vi "3458A Check Digitizing Process Status.vi"(5 "merge process exit error with main (True)":bool=TRUE, 7 "wait for exit (False)":bool, 8 "error in":errorcluster, 10 "channel id":i32, 11 "digitizer session in":T1 {"channels"."Range [Vpk]" min=0.0}) -> (0 "error out":errorcluster, 1 "proc error out":errorcluster, 2 "process exited?":bool, 3 "digitizer session out":T1 {"channels"."Range [Vpk]" min=0.0}, 4 "aux data out":T12, 6 "aux data valid?":bool)   [LabVIEW 2013, in "3458A Virtual Digitizer.lvlib"]
doc: "Checks execution status of digitizing process number 'channel id'. 'wait for exit' options specifies whether VI is just checking status or waits with timeout (3 seconds). If process exited and the 'wait for exit' is True the returned value from the process is returned in 'aux data out'. Exit status is returned in 'process exited' output. Once process exit value was returned, calling this VI will return error and invalid data!"
uses:
  3458A Virtual Digitizer.lvlib
  3458A Digitizer Session.ctl
  3458A Virtual Channel Config.ctl
  Counter/Counter Session.ctl
  Counter/Counter Type.ctl
  AWG/AWG Session.ctl
  AWG/AWG Type.ctl
  3458A Sync Mode.ctl
  3458A Idn Mode.ctl
  3458A Digitizing Low Levels/Configure/Sampling Mode.ctl
  3458A Digitizing Process Options.ctl
  3458A Data Packet.ctl
  3458A Aux Record Data.ctl
  3458A Digitizing Low Levels/Configure/Level Setup.ctl
  3458A Digitizing Low Levels/Configure/First Sample Trigger.ctl
  3458A Aperture Selection Mode.ctl
  Counter/Counter.lvlib
  AWG/AWG.lvlib
  3458A Digitizing Low Levels/3458A Digitizing Low Levels.lvlib
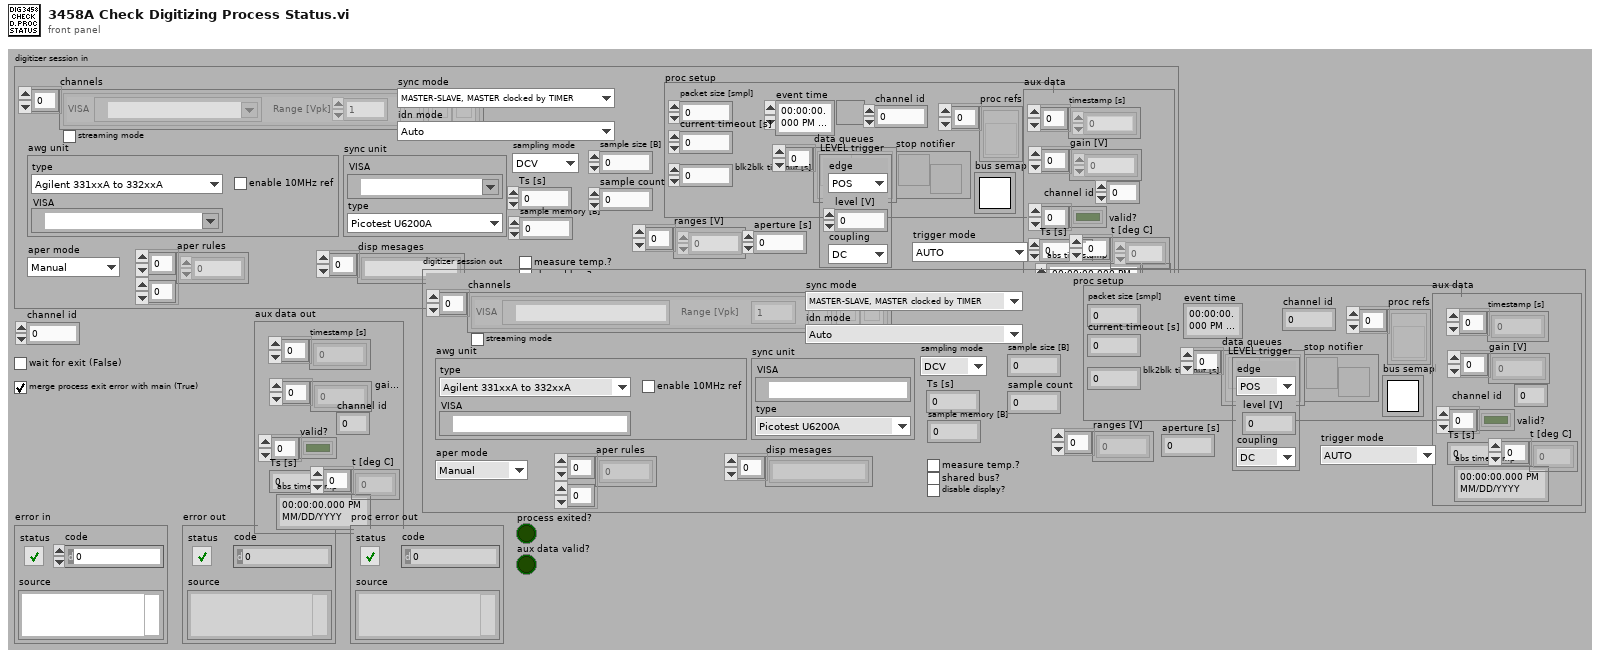
[diagram p1: front panel]
types:
  T1 = typedef "3458A Virtual Digitizer.lvlib/3458A Digitizer Session.ctl" = cluster{"channels":T2[], "sync unit":T3, "awg unit":T5, "sync mode":T7, "streaming mode":bool, "idn mode":T8, "sampling mode":T9, "Ts [s]":dbl, "sample memory [B]":i32, "proc setup":T10, "sample size [B]":i32, "sample count":i32, "aux data":T12, "ranges [V]":dbl[], "aperture [s]":dbl, "LEVEL trigger":T13, "trigger mode":T14, "measure temp.?":bool, "disp mesages":string[], "shared bus?":bool, "disable display?":bool, "aper mode":T15, "aper rules":dbl[][]}
  T2 = typedef "3458A Virtual Digitizer.lvlib/3458A Virtual Channel Config.ctl" = cluster{"VISA":refnum<visa-resource-name>, "Range [Vpk]":dbl, "btn clr":bool, "btn up":bool, "btn down":bool}
  T3 = typedef "Counter.lvlib/Counter Session.ctl" = cluster{"VISA":refnum<visa-resource-name>, "type":T4}
  T4 = typedef "Counter.lvlib/Counter Type.ctl" = enum16{"Picotest U6200A", "dummy"}
  T5 = typedef "AWG.lvlib/AWG Session.ctl" = cluster{"type":T6, "VISA":refnum<visa-resource-name>, "enable 10MHz ref":bool}
  T6 = typedef "AWG.lvlib/AWG Type.ctl" = enum16{"Agilent 331xxA to 332xxA", "Agilent 335xxA to 336xxA", "Tektronix AFG3101C", "dummy"}
  T7 = typedef "3458A Virtual Digitizer.lvlib/3458A Sync Mode.ctl" = enum16{"MASTER-SLAVE, MASTER clocked by TIMER", "MASTER-SLAVE, MASTER clocked by AWG", "ALL clocked by AWG", "MASTER-SLAVE, ALL clocked by TIMER", "ALL clocked by AWG with DFLL"}
  T8 = typedef "3458A Virtual Digitizer.lvlib/3458A Idn Mode.ctl" = enum16{"Auto", "Sequential (chn A, chn B, ...)", "From calibration string"}
  T9 = typedef "3458A Virtual Digitizer.lvlib/3458A Digitizing Low Levels.lvlib/Sampling Mode.ctl" = enum16{"DCV", "DSDC", "DSAC"}
  T10 = typedef "3458A Virtual Digitizer.lvlib/3458A Digitizing Process Options.ctl" = cluster{"channel id":i32, "packet size [smpl]":i32, "current timeout [s]":dbl, "blk2blk timeout [s]":dbl, "event time":timestamp, "stop notifier":refnum<notifier>, "data queues":refnum<queue>[], "proc refs":refnum<vi>[], "bus semaphore":T11}
  T11 = typedef "Semaphore RefNum" = refnum<k1>
  T12 = typedef "3458A Virtual Digitizer.lvlib/3458A Aux Record Data.ctl" = cluster{"channel id":i32, "valid?":bool[], "gain [V]":dbl[], "timestamp [s]":dbl[], "Ts [s]":dbl, "abs timestamp":timestamp, "t [deg C]":dbl[]}
  T13 = typedef "3458A Virtual Digitizer.lvlib/3458A Digitizing Low Levels.lvlib/Level Setup.ctl" = cluster{"edge":enum16{"POS", "NEG"}, "level [V]":dbl, "coupling":enum16{"DC", "AC"}}
  T14 = typedef "3458A Virtual Digitizer.lvlib/3458A Digitizing Low Levels.lvlib/First Sample Trigger.ctl" = enum16{"AUTO", "EXT", "SYN", "SGL", "HOLD", "LEVEL"}
  T15 = typedef "3458A Virtual Digitizer.lvlib/3458A Aperture Selection Mode.ctl" = enum16{"Manual", "Maximum", "Table"}
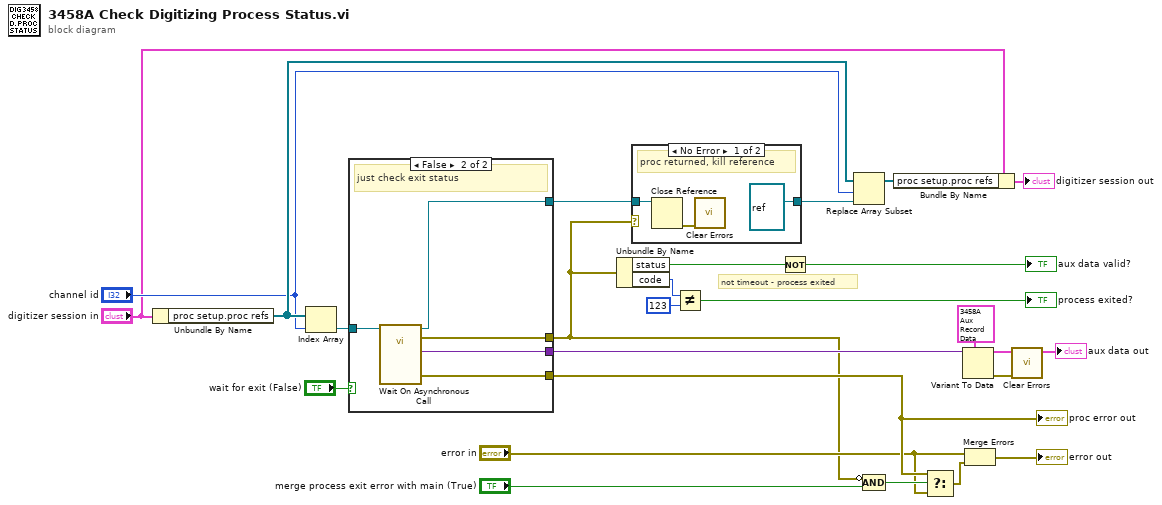
[diagram p0: block diagram]
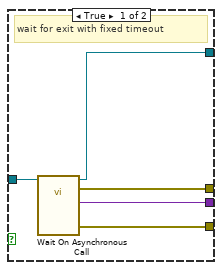
[diagram p3: hidden frame]
diagram:
  # "not timeout - process exited"
  n1 = Unbundle By Name("digitizer session in") -> ("proc setup.proc refs"=w15:refnum<vi>[])
  n2 = Index Array(array=w15, index="channel id") -> (element=w10:refnum<vi>)
  n3 = case shown="False" "wait for exit (False)" {
    tunnel: w10 -> [w28 w34]
    tunnel: [w30 w32] -> w16
    tunnel: [w29 w33] -> w25
    tunnel: [w27 w31] -> w1
    tunnel: [w26 w35] -> w7
    frame True {
      # "wait for exit with fixed timeout"
      n4 = call-by-ref "Wait On Asynchronous Call"(reference=w28) -> (reference out=w26:refnum<vi>, error out=w27:errorcluster, 0:"error out"=w30:errorcluster, "aux data out"=w29:variant)  [unwired: 11 in]
    }
    frame False {
      # "just check exit status"
      n5 = call-by-ref "Wait On Asynchronous Call"(reference=w34) -> (reference out=w35:refnum<vi>, error out=w31:errorcluster, 0:"error out"=w32:errorcluster, "aux data out"=w33:variant)  [unwired: 11 in]
    }
  }
  "proc error out" <- w16
  n6 = Unbundle By Name(w1) -> ("status"=w3:bool, "code"=w6:i32)
  n7 = case shown="No Error" w1 {
    tunnel: [refnum<vi> refnum ("proc ref") w39] -> w8
    tunnel: w7 -> [w36 w39]
    frame No Error {
      # "proc returned, kill reference"
      n8 = Close Reference(reference=w36) -> (error out=w38:errorcluster)  [unwired: 1 in]
      n9 = call <vilib>:"Clear Errors.vi"("error in (no error)"=w38) -> ()  [unwired: 6 in, 1 out]
    }
    frame Error {
    }
  }
  n10 = Not Equal?(x=w6, y=123) -> (x != y?=→"process exited?":bool)
  n11 = Not(x=w3) -> (.not. x?=→"aux data valid?":bool)
  n12 = Replace Array Subset(array=w15, new element=w8, index="channel id") -> (w12:refnum<vi>[])
  n13 = Compound Arithmetic op=AND(invert w1, "merge process exit error with main (True)") -> (w20:bool)
  n14 = Bundle By Name(cluster="digitizer session in", "proc setup.proc refs"=w12) -> (→"digitizer session out":T1)
  n15 = Select(t=w16, s=w20, f="error in") -> (s? t:f=w21:errorcluster)
  n16 = Variant To Data(type=T12 {"channel id"=0, "valid?"=[], "gain [V]"=[], "timestamp [s]"=[], "Ts [s]"=0.0, "abs timestamp"=timestamp(0 s since 1904-01-01), "t [deg C]"=[]} ("aux data"), Variant=w25) -> (data=→"aux data out":T12, error out=w23:errorcluster)  [unwired: 1 in]
  n17 = Merge Errors("error in", w21) -> (→"error out":errorcluster)
  n18 = call <vilib>:"Clear Errors.vi"("error in (no error)"=w23) -> ()  [unwired: 6 in, 1 out]
